vi "Robcomm_Run.vi"(2 "Program name":string="LDP1", 3 "DDE Service name":string="ROBCOMM") -> (1 "Error?":bool)   [LabVIEW 2012]
panel:
  out "Command":string="RUN"
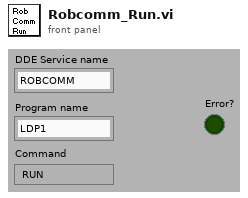
[diagram p1: front panel]
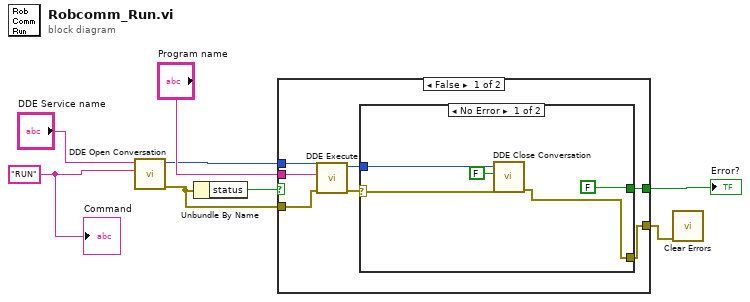
[diagram p0: block diagram]
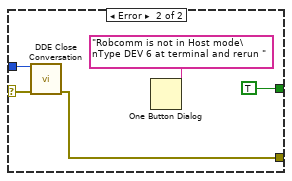
[diagram p2: hidden frame]
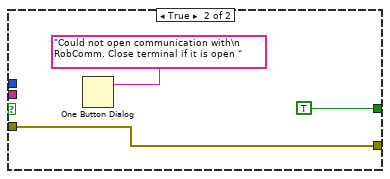
[diagram p3: hidden frame]
diagram:
  w5 = "RUN" ("topic")
  n1 = call <vilib>:"DDE Open Conversation.vi"("topic"=w5, "service"="DDE Service name") -> ("error out"=w2:errorcluster, "conversation refnum"=w6:u32)  [unwired: 6 in]
  n2 = Unbundle By Name(w2) -> ("status"=w1:bool)
  n3 = case shown="False" w1 {
    tunnel: w6 -> [w15 _]
    tunnel: "Program name" -> [w13 _]
    tunnel: w2 -> [w12 w27]
    tunnel: [w11 TRUE] -> w4
    tunnel: [w10 w27] -> w3
    frame False {
      n4 = call <vilib>:"DDE Execute.vi"("error in (no error)"=w12, "command"=w13, "conversation refnum in"=w15) -> ("error out"=w9:errorcluster, "conversation refnum out"=w14:u32)  [unwired: 5 in]
      n5 = case shown="No Error" w9 {
        selector: w9 -> [w19 w25]
        tunnel: w14 -> [w20 w24]
        tunnel: [FALSE TRUE] -> w11
        tunnel: [w17 w23] -> w10
        frame No Error {
          n6 = call <vilib>:"DDE Close Conversation.vi"("error in (no error)"=w19, "mode(T,close immediately)"=FALSE, "conversation refnum"=w20) -> ("error out"=w17:errorcluster)  [unwired: 6 in]
        }
        frame Error {
          n7 = call <vilib>:"DDE Close Conversation.vi"("error in (no error)"=w25, "conversation refnum"=w24) -> ("error out"=w23:errorcluster)  [unwired: 7 in]
          n8 = One Button Dialog(message="Robcomm is not in Host mode\nType DEV 6 at terminal and rerun ") -> ()  [unwired: 1 in, 1 out]
        }
      }
    }
    frame True {
      n9 = One Button Dialog(message="Could not open communication with\n RobComm. Close terminal if it is open ") -> ()  [unwired: 1 in, 1 out]
    }
  }
  "Error?" <- w4
  n10 = call <vilib>:"Clear Errors.vi"("error in (no error)"=w3) -> ()  [unwired: 6 in, 1 out]
  "Command" <- w5
